vi "Flatten Config.vi"(8 "error in (no error)":errorcluster, 10 "Configuration Data":T1, 11 "selected path":path) -> (0 "error out":errorcluster)   [LabVIEW 2013, in "About Screen Library.lvlib"]
uses:
  About Screen Library.lvlib
  Controls/Configuration Data.ctl
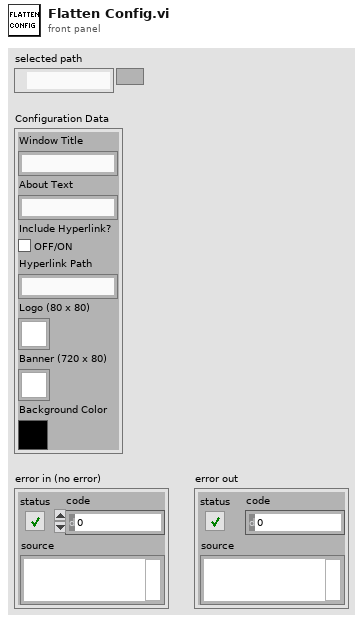
[diagram p1: front panel]
types:
  T1 = typedef "About Screen Library.lvlib/Configuration Data.ctl" = cluster{"Window Title":string, "About Text":string, "Include Hyperlink?":bool, "Hyperlink Path":string, "Logo (80 x 80)":picture, "Banner (720 x 80)":picture, "Background Color":u32}
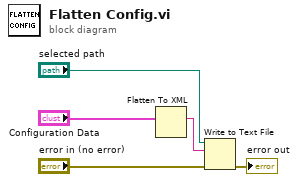
[diagram p0: block diagram]
diagram:
  n1 = Flatten To XML(anything="Configuration Data") -> (xml string=w2:string)
  n2 = Write to Text File(file (use dialog)="selected path", text=w2, error in="error in (no error)") -> (error out=→"error out":errorcluster)  [unwired: 1 in, 2 out]
